vi "Waveform Writing Example.vi"() -> ()   [LabVIEW 2014]
panel:
  in  "File Format":enum16{"CSV", "Binary", "HDF5", "TDMS"}(ring)
  out "Time Stamp":timestamp
  in  "Dataset (HDF5) or Group (TDMS)":string="MyData"
  in  "File Path":path
  in  "Comment":string="Testing file writing"
  in  "tf (s)":dbl=3600.0
  out "XY Graph":cluster{dbl[], dbl[]}[](graph)
  in  "Tf":dbl=5.0
  in  "T0":dbl=95.0
  in  "dt":dbl=0.1
  in  "k":dbl=0.0009
  # "Cooling Params"
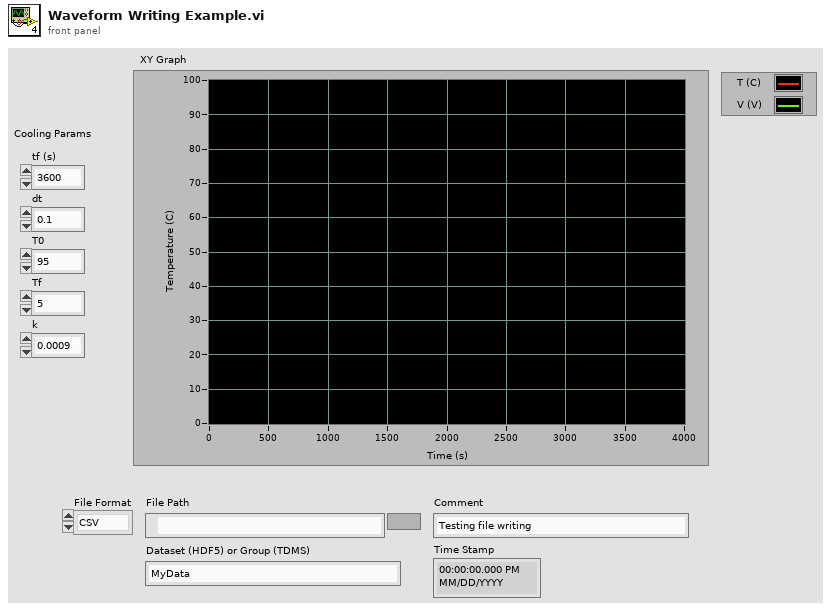
[diagram p1: front panel]
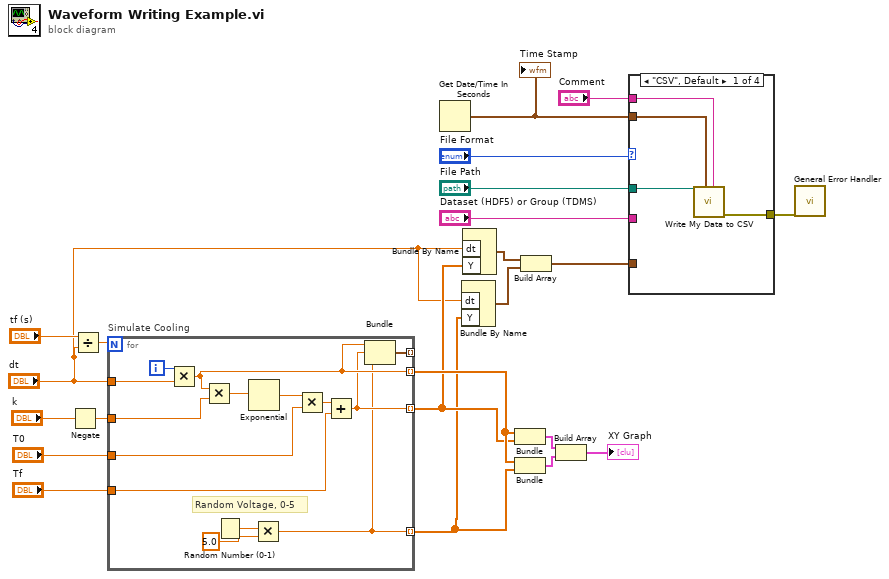
[diagram p0: block diagram]
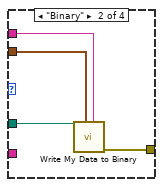
[diagram p2: hidden frame]
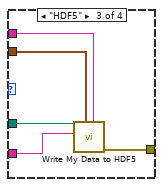
[diagram p3: hidden frame]
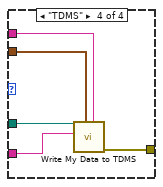
[diagram p4: hidden frame]
diagram:
  n1 = Negate(x="k") -> (-x=w16:dbl)
  n2 = Divide(x="tf (s)", y="dt") -> (x/y=w17:dbl)
  n3 = for "Simulate Cooling" {
    N: w17 -> [_]
    tunnel: "dt" -> [w32]
    tunnel: w16 -> [w31]
    tunnel: "T0" -> [w30]
    tunnel: "Tf" -> [w29]
    tunnel: [w26] -> w15 mode=indexing
    tunnel: [w25] -> w6 mode=indexing
    tunnel: [w24] -> w5 mode=indexing
    tunnel: [w23] -> _ mode=indexing
    i -> [w36]
    # "Random Voltage, 0-5"
    n4 = Multiply(x=w36, y=w32) -> (x*y=w26:dbl)
    n5 = Multiply(x=w26, y=w31) -> (x*y=w35:dbl)
    n6 = Random Number (0-1)() -> (number: 0 to 1=w28:dbl)
    n7 = Exponential(1:w35) -> (0:w34:dbl)
    n8 = Multiply(x=w28, y=5.0) -> (x*y=w24:dbl)
    n9 = Multiply(x=w34, y=w30) -> (x*y=w33:dbl)
    n10 = Add(x=w33, y=w29) -> (x+y=w25:dbl)
    n11 = Bundle(w26, w25, w24) -> (w23:cluster{dbl, dbl, dbl})  [unwired: 1 in]
  }
  n12 = Get Date/Time In Seconds() -> (seconds since 1Jan1904=w10:timestamp)
  "Time Stamp" <- w10
  n13 = Bundle By Name("dt"="dt", "Y"=w5) -> (w2:waveform(dbl))  [unwired: 1 in]
  n14 = Bundle By Name("dt"="dt", "Y"=w6) -> (w3:waveform(dbl))  [unwired: 1 in]
  n15 = Bundle(w15, w6) -> (w14:cluster{dbl[], dbl[]})  [unwired: 1 in]
  n16 = Bundle(w15, w5) -> (w13:cluster{dbl[], dbl[]})  [unwired: 1 in]
  n17 = Build Array(w3, w2) -> (w1:waveform(dbl)[])
  n18 = Build Array(w14, w13) -> (→"XY Graph":cluster{dbl[], dbl[]}[])
  n19 = case shown="\"CSV\", Default" "File Format" {
    tunnel: "File Path" -> [w40 w44 w49 w54]
    tunnel: w10 -> [w39 w43 w48 w53]
    tunnel: "Comment" -> [w38 w42 w47 w52]
    tunnel: w1 -> [_ _ _ _]
    tunnel: [w37 w41 w46 w51] -> w8
    tunnel: "Dataset (HDF5) or Group (TDMS)" -> [_ _ w45 w50]
    frame "CSV", Default {
      n20 = call "Write My Data to CSV.vi"("Comment"=w38, "Time Stamp"=w39, "file path"=w40) -> ("error out"=w37:errorcluster)  [unwired: 8 in]
    }
    frame "Binary" {
      n21 = call "Write My Data to Binary.vi"("Comment"=w42, "Time Stamp"=w43, "file path"=w44) -> ("error out"=w41:errorcluster)  [unwired: 8 in]
    }
    frame "HDF5" {
      n22 = call "Write My Data to HDF5.vi"("Comment"=w47, "Time Stamp"=w48, "Dataset Path"=w45, "file path"=w49) -> ("error out"=w46:errorcluster)  [unwired: 7 in]
    }
    frame "TDMS" {
      n23 = call "Write My Data to TDMS.vi"("Comment"=w52, "Time Stamp"=w53, "Dataset Path"=w50, "file path"=w54) -> ("error out"=w51:errorcluster)  [unwired: 7 in]
    }
  }
  n24 = call <vilib>:"General Error Handler.vi"("error in (no error)"=w8) -> ()  [unwired: 10 in, 5 out]
